vi "BinGeneration.vi"() -> ()   [LabVIEW 2015]
panel:
  in  "file path (use dialog)":path=path "C:/Users/leser/Documents/LabVIEW Data/Apps/Lab Exercises/Prueba8.bin"
  out "Array":dbl[](array[numeric])=[0.1470064516231846, 0.8997285083084419, 0.4252961467219172, 0.33109142347701503, 0.5520000454429304, 0.9196285157615773, 0.5824842556440388, 0.4689799785044455, 0.2668038833024986, 0.5863081870844116, 0.8575702791951654, 0.8954336330353123, 0.9651717297905247, 0.6027272527926352, 0.38712188164182537, 0.4092776218998022, 0.2267719374782775, 0.575540024927971, 0.844737205645708, 0.5863886511374197, 0.9264652331940029, 0.9091263176505024, 0.7098478537295401, 0.9976913684927187, 0.49555239091159775, 0.39871146842177135, 0.44226608633136766, 0.8917230180310751, 0.27885068325515405, 0.4461130791342782, 0.2754491845235807, 0.944206943924637, 0.664992011224153, 0.3599520850112876, 0.7141119462601526, 0.27842828564879163, 0.32870054338845955, 0.6330836885440361, 0.06824048463195176, 0.5050061890453765, 0.6424498178175755, 0.5766202463173467, 0.9687422123713583, 0.47058808628239657, 0.7037312076394466, 0.8975499409827592, 0.9890586101494088, 0.6985896553170994, 0.7840050862326893, 0.12595696042770266]
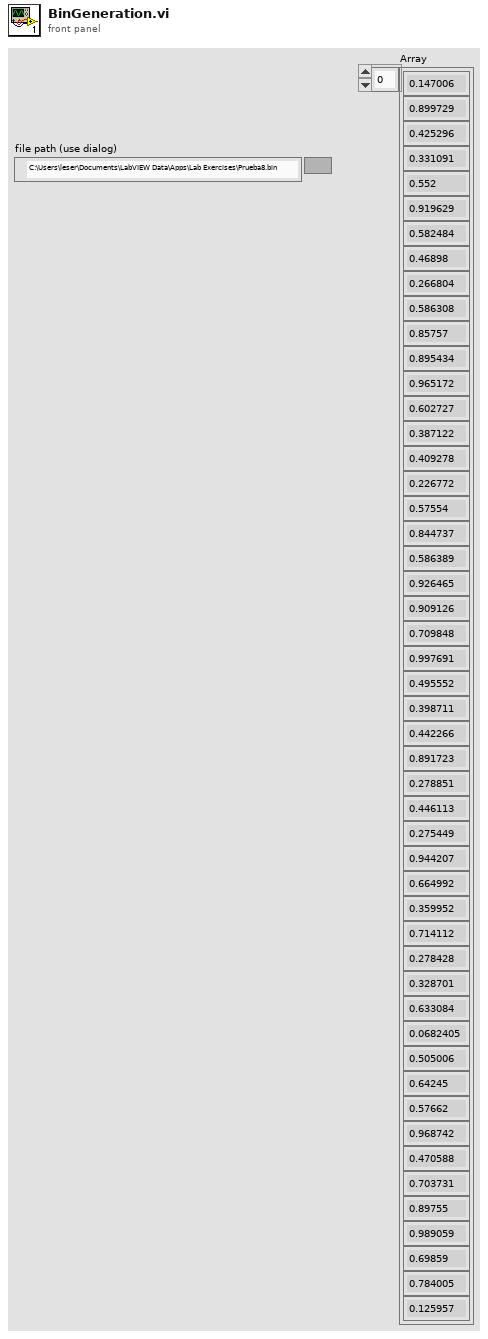
[diagram p1: front panel]
types:
  T1 = enum16{"big-endian, network order", "native, host order", "little-endian"}
  T2 = enum16{"open", "replace", "create", "open or create", "replace or create", "replace or create with confirmation"}
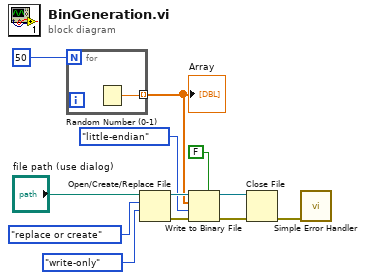
[diagram p0: block diagram]
diagram:
  n1 = for {
    N: 50 -> [_]
    tunnel: [w13] -> w7 mode=indexing
    n2 = Random Number (0-1)() -> (number: 0 to 1=w13:dbl)
  }
  "Array" <- w7
  n3 = Open/Create/Replace File(file path (use dialog)="file path (use dialog)", operation (0:open)=T2."replace or create", access (0:read/write)=enum16{"read/write", "read-only", "write-only"}."write-only") -> (refnum out=w8:refnum<file>, error out=w5:errorcluster)  [unwired: 3 in, 1 out]
  n4 = Write to Binary File(file (use dialog)=w8, data=w7, error in=w5, 5:FALSE ("prepend array or string size? (T)"), 9:T1."little-endian" ("byte order (0:big-endian, network order)")) -> (refnum out=w3:refnum<file>, error out=w4:errorcluster)  [unwired: 1 in, 1 out]
  n5 = Close File(refnum=w3, error in=w4) -> (error out=w1:errorcluster)  [unwired: 1 out]
  n6 = call <vilib>:"Simple Error Handler.vi"("error in (no error)"=w1) -> ()  [unwired: 4 in, 5 out]
